vi "AutoDistancePID.vi"(10 "DesiredDistance":dbl format="%.2f", 11 "ActualDistance":dbl format="%.2f") -> (1 "TankDriveRight":dbl format="%.2f", 2 "TankDriveLeft":dbl format="%.2f")   [LabVIEW 2013]
doc: "Uses a PID to move the robot from the actual distance to the desired distance. Returns values for tank drive left and tank drive right that can be fed directly into tank drive."
uses:
  <vilib>/addons/control/pid/pid.llb/PID (DBL).vi
  <vilib>/addons/control/pid/NI_PID_pid.lvlib
panel:
  in  "reinitialize? (F)":bool
  in  "PID gains":T1={"proportional gain (Kc)"=1.0, "integral time (Ti, min)"=0.0, "derivative time (Td, min)"=0.0} {"derivative time (Td, min)" format="%.3f"; "integral time (Ti, min)" format="%.3f"; "proportional gain (Kc)" format="%.3f"}
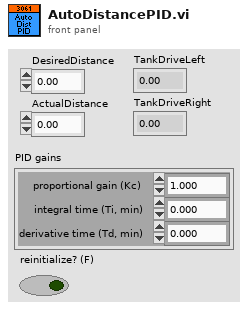
[diagram p1: front panel]
types:
  T1 = cluster{"proportional gain (Kc)":dbl, "integral time (Ti, min)":dbl, "derivative time (Td, min)":dbl}
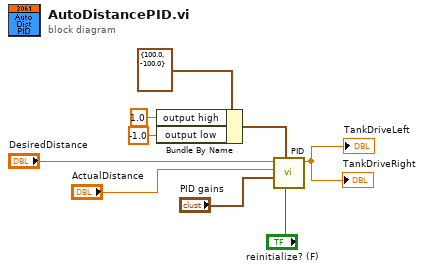
[diagram p0: block diagram]
diagram:
  n1 = Bundle By Name(cluster=cluster{"output high":dbl, "output low":dbl} {"output high"=100.0, "output low"=-100.0} ("output range"), "output high"=1.0, "output low"=-1.0) -> (w6:cluster{"output high":dbl, "output low":dbl})
  n2 = call-poly <vilib>:"PID.vi"("reinitialize? (F)"="reinitialize? (F)", "output range"=w6, "PID gains"="PID gains", "process variable"="ActualDistance", "setpoint"="DesiredDistance") -> ("output"=→"TankDriveLeft" →"TankDriveRight":dbl)  [unwired: 5 in, 1 out]
